vi "ScopeInitSubVI.vi"() -> (0 "instrument handle out":refnum<k15>)   [LabVIEW 2012]
uses:
  <instrlib>/niScope/Controls/niScope vertical coupling.ctl
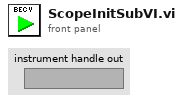
[diagram p1: front panel]
types:
  T1 = typedef "niScope vertical coupling.ctl" = i32
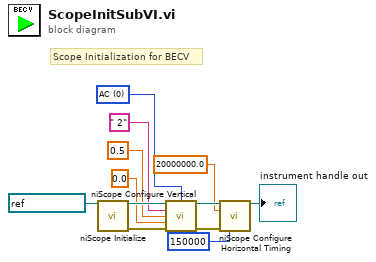
[diagram p0: block diagram]
diagram:
  w3 = T1 0 items=["AC", "DC", "Ground"] ("vertical coupling")
  # "Scope Initialization for BECV"
  n1 = call <instrlib>:"niScope Initialize.vi"("resource name"=refnum<k15> "PXI1Slot4") -> ("instrument handle"=w12:refnum<k15>, "error out"=w11:errorcluster)  [unwired: 13 in]
  n2 = call <instrlib>:"niScope Configure Vertical.vi"("instrument handle"=w12, "vertical coupling"=w3, "channels"=" 2", "vertical range"=0.5, "vertical offset"=0.0, "error in"=w11) -> ("instrument handle out"=w9:refnum<k15>, "error out"=w8:errorcluster)  [unwired: 8 in]
  n3 = call <instrlib>:"niScope Configure Horizontal Timing.vi"("instrument handle"=w9, "min sample rate"=20000000.0, "error in"=w8, "min record length"=150000) -> ("instrument handle out"=→"instrument handle out":refnum<k15>)  [unwired: 10 in, 1 out]
